vi "Test Sync.vi"(8 "error in (no error)":errorcluster, 11 "SR7270 Drivers in":refnum<class "SR7270 Drivers.lvclass">) -> (0 "error out":errorcluster, 3 "SR7270 Drivers out":refnum<class "SR7270 Drivers.lvclass">)   [LabVIEW 2016, in "SR7270 Drivers.lvlib" / "SR7270 Drivers.lvclass"]
uses:
  SR7270 Drivers.lvclass
  Typedefs/SYNC--enum.ctl
  SR7270 Drivers.lvclass/SR7270 Drivers.ctl
  <vilib>/addons/_JKI Toolkits/Caraya/classes/Assert/Assert.lvclass
  <vilib>/addons/_JKI Toolkits/Caraya/classes/Test/Test.lvclass
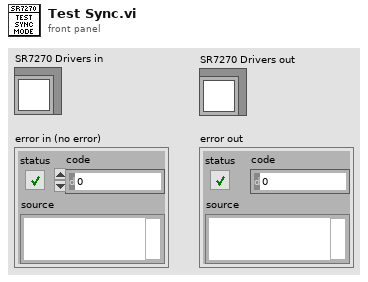
[diagram p1: front panel]
types:
  T1 = typedef "SR7270 Drivers.lvlib/SR7270 Drivers.lvclass/SYNC--enum.ctl" = enum16{"Disabled", "Enabled"}
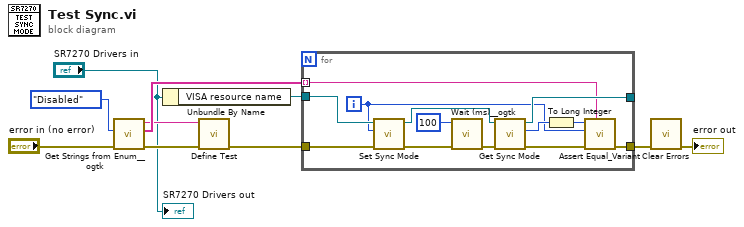
[diagram p0: block diagram]
diagram:
  n1 = call <userlib>:"Get Strings from Enum__ogtk.vi"("error in (no error)"="error in (no error)", "Enum"=SYNC--enum."Disabled" ("Synchronous Time Constant Mode")) -> ("error out"=w5:errorcluster, "Enum Strings"=w8:string[], "Enum Name"=w6:string)  [unwired: 6 in, 1 out]
  n2 = Unbundle By Name("SR7270 Drivers in") -> ("VISA resource name"=w2:refnum<visa-resource-name>)
  n3 = call <vilib>:"Define Test.vi"("error in (no error)"=w5, "Label (VI Title)"=w6) -> ("error out"=w3:errorcluster)  [unwired: 9 in]
  n4 = for {
    tunnel: w2 -> [w22]
    tunnel: w3 -> [w14]
    tunnel: [w20] -> w10
    tunnel: [w19] -> _
    tunnel: w8 -> [w11] mode=indexing
    i -> [w13]
    n5 = call "Set Sync Mode.vi"("error in (no error)"=w14, "Synchronous Time Constant Mode"=w13, "VISA resource name"=w22) -> ("error out"=w16:errorcluster, "VISA resource name out"=w23:refnum<visa-resource-name>)  [unwired: 7 in]
    n6 = call <userlib>:"Wait (ms)__ogtk.vi"("error in (no error)"=w16, "milliseconds to wait"=u32 100) -> ("error out"=w18:errorcluster)  [unwired: 8 in, 1 out]
    n7 = call "Get Sync Mode.vi"("error in (no error)"=w18, "VISA resource name"=w23) -> ("error out"=w21:errorcluster, "Synchronous Time Constant Mode"=w15:T1, "VISA resource name out"=w19:refnum<visa-resource-name>)  [unwired: 7 in]
    n8 = To Long Integer(number=w15) -> (32bit integer=w12:i32)
    n9 = call <vilib>:"Assert Equal_Variant.vi"("Label"=w11, "error in (no error)"=w21, "Y"=w13, "X"=w12) -> ("error out"=w20:errorcluster)  [unwired: 7 in]
  }
  n10 = call <vilib>:"Clear Errors.vi"("error in (no error)"=w10) -> ("error out"=→"error out":errorcluster)  [unwired: 5 in, 1 out]
  "SR7270 Drivers out" <- "SR7270 Drivers in"
